vi "Ophir BuildFrame.vi"(2 "error in (no error)":errorcluster, 3 "Command Input":string) -> (0 "error out":errorcluster, 1 "Output Frame":string)   [LabVIEW 2017]
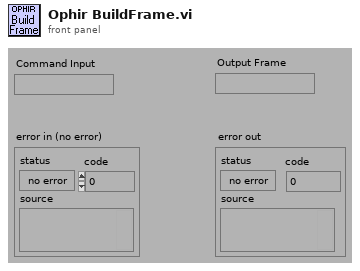
[diagram p1: front panel]
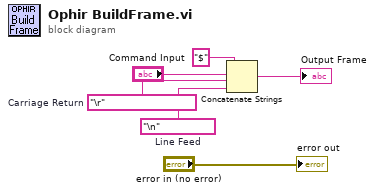
[diagram p0: block diagram]
diagram:
  w3 = "\n"  # Line Feed
  w4 = "\r"  # Carriage Return
  n1 = Concatenate Strings("$", "Command Input", w4, w3) -> (→"Output Frame":string)
  "error out" <- "error in (no error)"
